vi "GetBandBounds.vi"(8 "error in (no error)":errorcluster, 11 "Properties In":T1[](array[typedef])) -> (0 "error out":errorcluster, 1 "High":sgl, 2 "Low":sgl, 3 "Properties Out":T1[](array[typedef]))   [LabVIEW 2015]
uses:
  <vilib>/addons/InsightCM/MessageBus/Base/controls/KeyValuePair.ctl
  <vilib>/addons/InsightCM/Utilities/PropertyHelpers/PropertyHelpers.lvlib
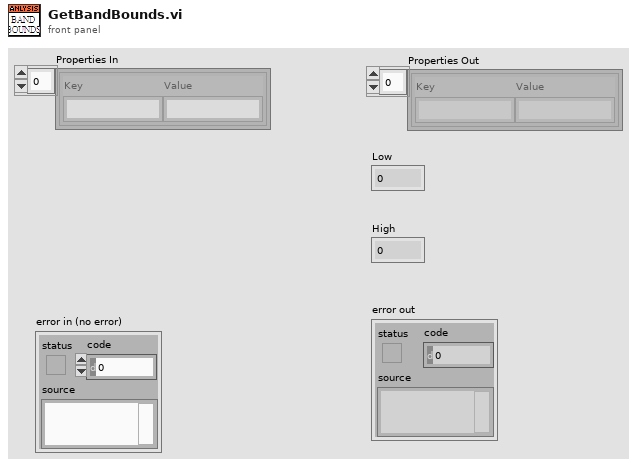
[diagram p1: front panel]
types:
  T1 = typedef "KeyValuePair.ctl" = cluster{"Key":string, "Value":string}
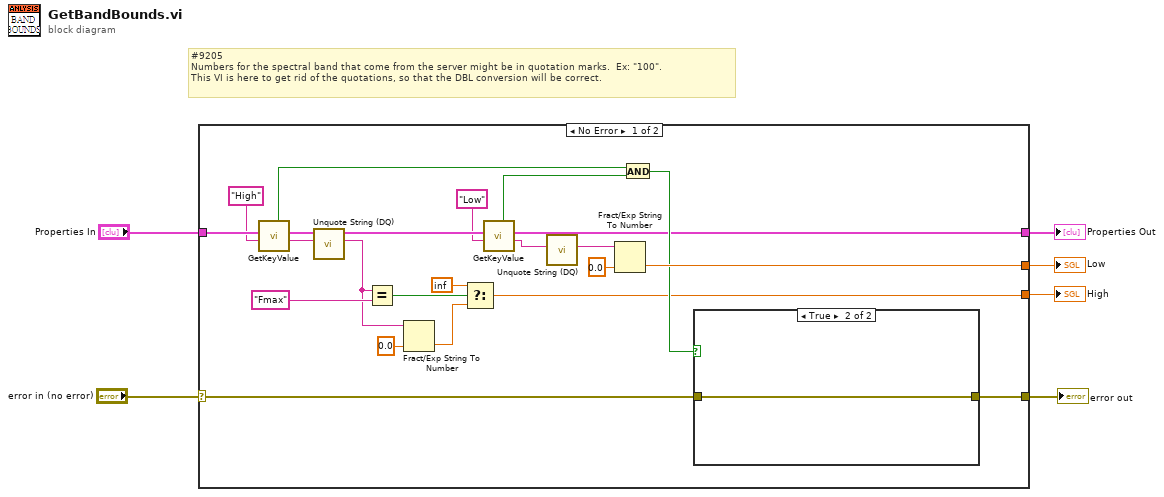
[diagram p0: block diagram]
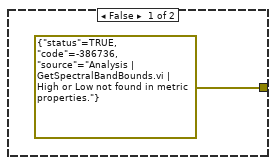
[diagram p2: hidden frame]
diagram:
  # "#9205\nNumbers for the spectral band that come from the server might be in quotation marks.  Ex: \"100\".\nThis VI is here to get rid of the quotations, so that the DBL conversion will be correct."
  n1 = case shown="No Error" "error in (no error)" {
    selector: "error in (no error)" -> [w22 w32]
    tunnel: [w21 w31] -> w6
    tunnel: [w11 _] -> w5
    tunnel: [w27 _] -> w4
    tunnel: "Properties In" -> [w20 w31]
    tunnel: [w23 w32] -> w1
    frame No Error {
      n2 = call <vilib>:"GetKeyValue.vi"("key"="High", "key value pairs"=w20) -> ("value"=w10:string, "key value pairs out"=w19:T1[], "found"=w25:bool)  [unwired: 7 in]
      n3 = call "Unquote String (DQ).vi"("Input String"=w10) -> ("Output String"=w9:string)  [unwired: 6 in]
      n4 = Equal?(x=w9, y="Fmax") -> (x = y?=w14:bool)
      n5 = Fract/Exp String To Number(string=w9, default (0 dbl)=sgl 0.0 ("default (0 DBL)")) -> (number=w12:sgl)  [unwired: 2 in, 1 out]
      n6 = Select(t=sgl inf, s=w14, f=w12) -> (s? t:f=w11:sgl)
      n7 = call <vilib>:"GetKeyValue.vi"("key"="Low", "key value pairs"=w19) -> ("value"=w8:string, "key value pairs out"=w21:T1[], "found"=w26:bool)  [unwired: 7 in]
      n8 = call "Unquote String (DQ).vi"("Input String"=w8) -> ("Output String"=w7:string)  [unwired: 6 in]
      n9 = Fract/Exp String To Number(string=w7, default (0 dbl)=sgl 0.0 ("default (0 DBL)")) -> (number=w27:sgl)  [unwired: 2 in, 1 out]
      n10 = And(x=w25, y=w26) -> (x .and. y?=w24:bool)
      n11 = case shown="True" w24 {
        tunnel: [errorcluster {"status"=TRUE, "code"=-386736, "source"="Analysis | GetSpectralBandBounds.vi | High or Low not found in metric properties."} ("error in") w30] -> w23
        tunnel: w22 -> [_ w30]
        frame False {
        }
        frame True {
        }
      }
    }
    frame Error {
    }
  }
  "High" <- w5
  "Low" <- w4
  "Properties Out" <- w6
  "error out" <- w1
